vi "Control Panel Refresh.vi"(11 "Data In":string[][](array[string]) caption="所有行") -> (2 "Data":T1(array[cluster]), 3 "Array":cluster{string[][]}[](array[cluster]))   [LabVIEW 2020]
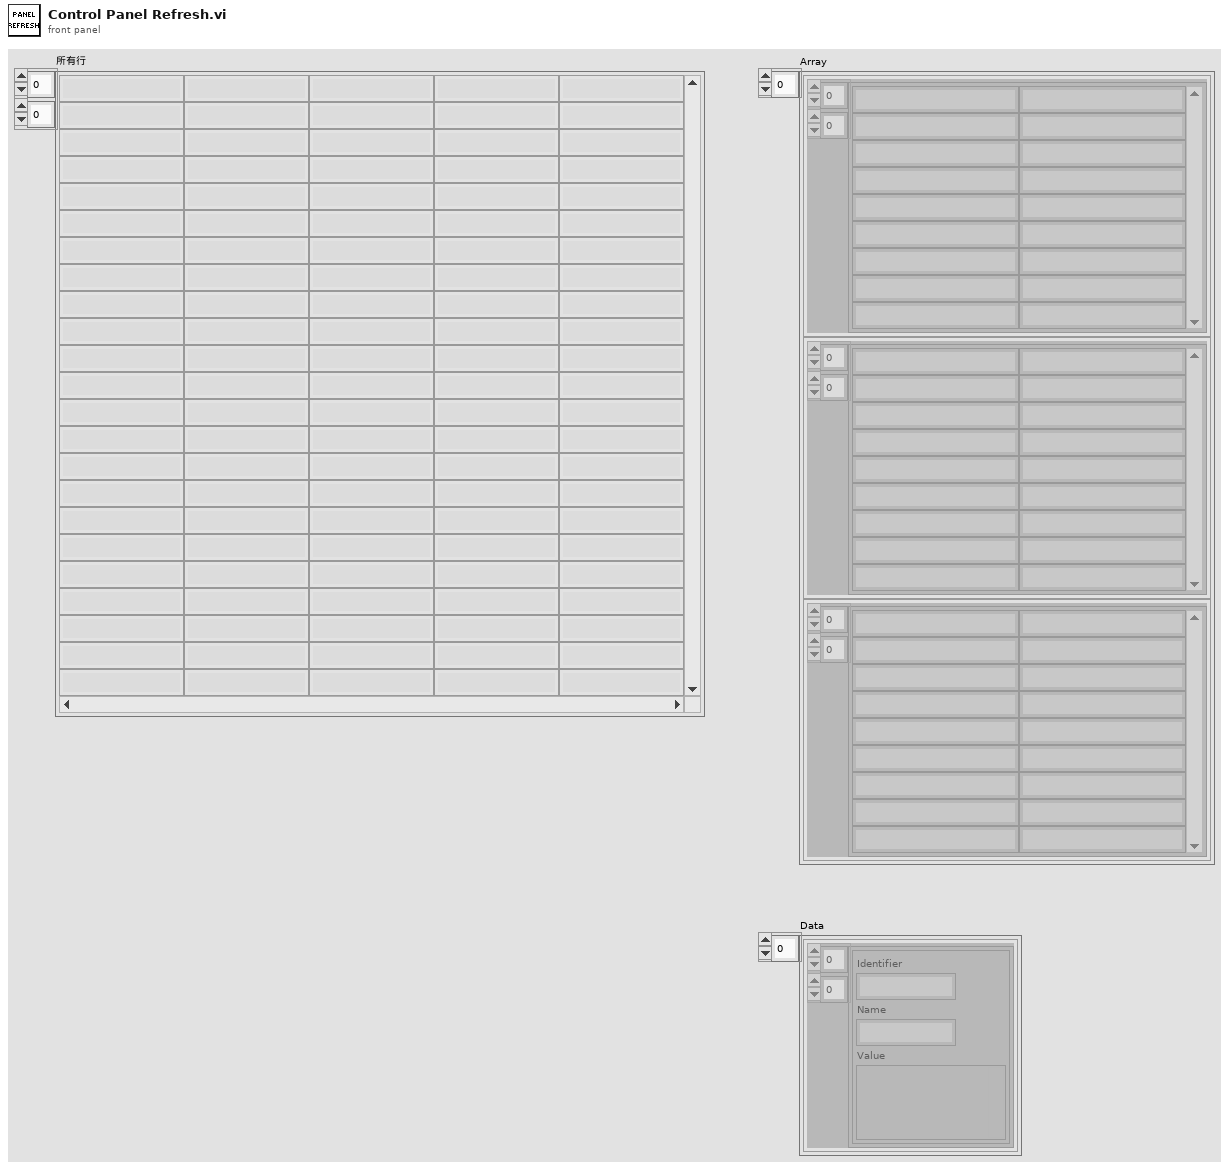
[diagram p1: front panel]
types:
  T1 = cluster{cluster{"Identifier":string, "Name":string, "Value":variant}[][]}[]
  T2 = map{string, map{string, cluster{"Module Name":string, "Name":string, "Index":string, "Identifier":string}}}
  T3 = map{string, cluster{"Module Name":string, "Name":string, "Index":string, "Identifier":string}}
  T4 = cluster{"Module Name":string, "Name":string, "Index":string, "Identifier":string}
  T5 = cluster{"Identifier":string, "Name":string, "Value":variant}
  T6 = cluster{"Identifier":string, "Name":string, "Value":variant}[]
  T7 = cluster{"Identifier":string, "Name":string, "Value":variant}[][]
  T8 = cluster{cluster{"Identifier":string, "Name":string, "Value":variant}[][]}
  T9 = typedef "LVRectTypeDef.ctl" = cluster{"Left":i16, "Top":i16, "Right":i16, "Bottom":i16}
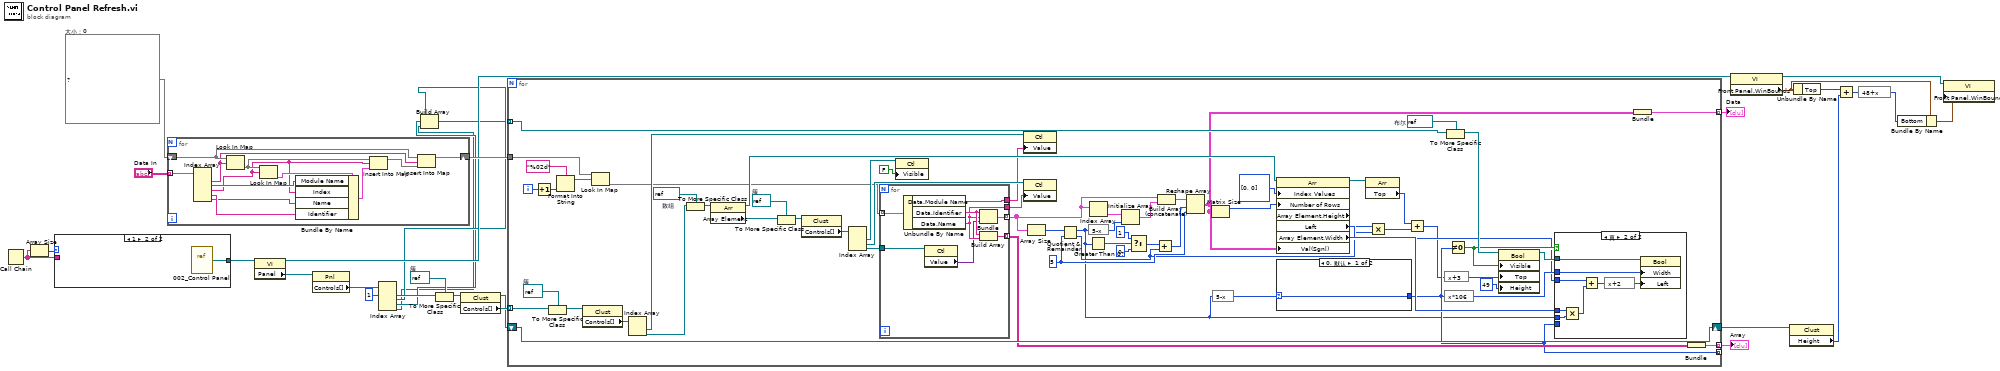
[diagram p0: block diagram]
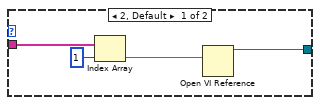
[diagram p4: hidden frame]
diagram:
  w19 = T2 {}  # 大小：0
  w24 = refnum<vi> refnum  # 簇
  n1 = Call Chain() -> (call chain=w28:string[])
  n2 = Array Size(array=w28) -> (size(s)=w29:i32)
  n3 = case shown="1" w29 {
    tunnel: w28 -> [w33 _]
    tunnel: [w30 w34] -> w27
    frame 2, Default {
      n4 = Index Array(array=w33, index=1 ("索引")) -> (element=w32:string)
      n5 = Open VI Reference(vi path=w32) -> (vi reference=w30:refnum<vi>)  [unwired: 5 in, 1 out]
    }
    frame 1 {
      n6 = vi-ref "002_Control Panel.vi"() -> (w34:refnum<vi>)
    }
  }
  n7 = for {
    tunnel: "Data In" -> [w44] mode=indexing
    shift-right: [w45] -> w18
    shift-left: w19 -> [w46]
    n8 = Index Array(array=w44) -> (element #1=w42:string, element #2=w38:string, element #3=w37:string, element #4=w36:string, element #5=w35:string)  [unwired: 5 in]
    n9 = Look In Map(map=w46, key=w42) -> (value=w41:T3)  [unwired: 1 in, 1 out]
    n10 = Look In Map(map=w41, key=w37) -> (value=w43:T4)  [unwired: 1 in, 1 out]
    n11 = Bundle By Name(cluster=w43, "Module Name"=w38, "Index"=w37, "Name"=w35, "Identifier"=w36) -> (w40:T4)
    n12 = Insert Into Map(map in=w41, key=w37, value=w40) -> (map out=w39:T3)  [unwired: 2 out]
    n13 = Insert Into Map(map in=w46, key=w42, value=w39) -> (map out=w45:T2)  [unwired: 2 out]
  }
  n14 = property class="VI"(reference=w27) -> (reference out=w17:refnum<vi>, "Panel"=w26:refnum<vi>)  [unwired: 1 in, 1 out]
  n15 = property class="Pnl"(reference=w26) -> ("Controls[]"=w25:refnum<vi>[])  [unwired: 1 in, 2 out]
  n16 = Index Array(array=w25, index #1=1 ("索引")) -> (element #1=w23:refnum<vi>, element #2=w5:refnum<vi>, element #3=w4:refnum<vi>, element #4=w3:refnum<vi>)  [unwired: 3 in]
  n17 = Build Array(w5, w4, w3) -> (w2:refnum<vi>[])
  n18 = To More Specific Class(target class=w24, reference=w23) -> (specific class reference=w22:refnum<vi>)  [unwired: 1 in, 1 out]
  n19 = property class="Clust"(reference=w22) -> (reference out=w10:refnum<vi>, "Controls[]"=w21:refnum<vi>[])  [unwired: 1 in, 1 out]
  n20 = for {
    tunnel: w21 -> [w109] mode=indexing
    tunnel: w18 -> [w54]
    shift-right: [w82] -> w9
    shift-left: w10 -> [w82]
    tunnel: [w80] -> w7 mode=indexing
    tunnel: w2 -> [w79] mode=indexing
    tunnel: [w68] -> _ mode=indexing
    tunnel: [w48] -> w1 mode=indexing
    i -> [w52]
    w77 = refnum<vi> refnum  # 布尔
    w88 = 5 ("y")
    w101 = refnum<vi> refnum  # 簇
    w104 = refnum<vi> refnum  # 数组
    w108 = refnum<vi> refnum  # 簇
    n21 = Increment(x=w52) -> (x+1=w51:i32)
    n22 = To More Specific Class(target class=w108, reference=w109) -> (specific class reference=w107:refnum<vi>)  [unwired: 1 in, 1 out]
    n23 = Format Into String(format string="%02d" ("格式字符串"), w51) -> (resulting string=w50:string)  [unwired: 2 in, 1 out]
    n24 = property class="Clust"(reference=w107) -> ("Controls[]"=w106:refnum<vi>[])  [unwired: 1 in, 2 out]
    n25 = Look In Map(map=w54, key=w50) -> (value=w49:T3)  [unwired: 1 in, 1 out]
    n26 = Index Array(array=w106) -> (element #1=w85:refnum<vi>, element #2=w103:refnum<vi>)  [unwired: 2 in]
    n27 = To More Specific Class(target class=w104, reference=w103) -> (specific class reference=w105:refnum<vi>)  [unwired: 1 in, 1 out]
    n28 = property class="Arr"(reference=w105) -> (reference out=w93:refnum<vi>, "Array Element"=w100:refnum<vi>)  [unwired: 1 in, 1 out]
    n29 = To More Specific Class(target class=w101, reference=w100) -> (specific class reference=w102:refnum<vi>)  [unwired: 1 in, 1 out]
    n30 = property class="Clust"(reference=w102) -> ("Controls[]"=w99:refnum<vi>[])  [unwired: 1 in, 2 out]
    n31 = Index Array(array=w99) -> (element #1=w98:refnum<vi>, element #2=w96:refnum<vi>, element #3=w95:refnum<vi>)  [unwired: 3 in]
    n32 = for {
      tunnel: w95 -> [w126]
      tunnel: [w121] -> w94
      tunnel: w49 -> [w125] mode=indexing
      tunnel: [w124] -> w58 mode=indexing
      tunnel: [w123] -> w84
      tunnel: [w120] -> w81 mode=indexing
      n33 = Unbundle By Name(w125) -> ("Data.Module Name"=w123:string, "Data.Identifier"=w122:string, "Data.Name"=w121:string)
      n34 = property class="Ctl"(reference=w126) -> ("Value"=w119:variant)  [unwired: 1 in, 2 out]
      n35 = Bundle("Identifier"=w122, "Name"=w121, "Value"=w119) -> (w124:T5)  [unwired: 1 in]
      n36 = Build Array(w122, w121) -> (w120:string[])
    }
    n37 = property class="Ctl"(reference=w98, "Visible"=FALSE ("可见")) -> ()  [unwired: 1 in, 2 out]
    n38 = property class="Ctl"(reference=w85, "Value"=w84) -> ()  [unwired: 1 in, 2 out]
    n39 = property class="Ctl"(reference=w96, "Value"=w94) -> ()  [unwired: 1 in, 2 out]
    n40 = Array Size(array=w58) -> (size(s)=w70:i32)
    n41 = Quotient & Remainder(x=w70, y=w88) -> (x-y*floor(x/y)=w61:i32, floor(x/y)=w66:i32)
    n42 = expression code="5-x"(w61) -> (w71:i32)
    n43 = Index Array(array=w58) -> (element=w87:T5)  [unwired: 1 in]
    n44 = Greater Than 0?(x=w61) -> (x > 0?=w90:bool)
    n45 = Initialize Array(w87, w71) -> (w57:T6)
    n46 = Select(t=1, s=w90, f=0) -> (s? t:f=w89:i32)
    n47 = Add(x=w89, y=w66) -> (x+y=w86:i32)
    n48 = Build Array (concatenate)(w58, w57) -> (w56:T6)
    n49 = Reshape Array(w56, w86, w88) -> (w47:T7)
    n50 = Matrix Size(0:w47) -> (1:w83:i32)  [unwired: 1 out]
    n51 = expression code="5-x"(w61) -> (w69:i32)
    n52 = property class="Arr"(reference=w93, "Index Values"=u32[] [0, 0] ("索引值"), "Number of Rows"=w83, "Val(Sgnl)"=w47) -> (reference out=w60:refnum<vi>, "Array Element.Height"=w65:u32, "Left"=w72:i32, "Array Element.Width"=w73:u32)  [unwired: 1 in, 1 out]
    n53 = case shown="0, 默认" w69 {
      selector: w69 -> [w110 _]
      tunnel: [w110 _] -> w68
      frame 0, Default {
      }
      frame 5.. {
      }
    }
    n54 = property class="Arr"(reference=w60) -> ("Top"=w59:i32)  [unwired: 1 in, 2 out]
    n55 = Multiply(x=w65, y=w66) -> (x*y=w64:u32)
    n56 = Add(x=w59, y=w64) -> (x+y=w63:u32)
    n57 = expression code="x*106"(w68) -> (w75:i32)
    n58 = expression code="x+3"(w63) -> (w62:u32)
    n59 = To More Specific Class(target class=w77, reference=w79) -> (specific class reference=w78:refnum<vi>)  [unwired: 1 in, 1 out]
    n60 = Not Equal To 0?(x=w68) -> (x != 0?=w74:bool)
    n61 = property class="Bool"(reference=w78, "Visible"=w74, "Top"=w62, "Height"=u32 49 ("按钮大小:高度")) -> (reference out=w76:refnum<vi>)  [unwired: 1 in, 1 out]
    n62 = case shown="真" w74 {
      tunnel: w76 -> [_ w118]
      tunnel: w75 -> [_ w117]
      tunnel: w68 -> [_ _]
      tunnel: w73 -> [_ w116]
      tunnel: w72 -> [_ w115]
      tunnel: w61 -> [_ w111]
      frame False {
      }
      frame True {
        n63 = Multiply(x=w116, y=w111) -> (x*y=w113:u32)
        n64 = Add(x=w115, y=w113) -> (x+y=w114:u32)
        n65 = expression code="x+2"(w114) -> (w112:u32)
        n66 = property class="Bool"(reference=w118, "Width"=w117, "Left"=w112) -> ()  [unwired: 1 in, 2 out]
      }
    }
    n67 = Bundle(w47) -> (w48:T8)  [unwired: 1 in]
    n68 = Bundle(w81) -> (w80:cluster{string[][]})  [unwired: 1 in]
  }
  "Array" <- w7
  "Data" <- w1
  n69 = property class="VI"(reference=w17) -> (reference out=w15:refnum<vi>, "Front Panel.WinBounds"=w14:T9)  [unwired: 1 in, 1 out]
  n70 = property class="Clust"(reference=w9) -> ("Height"=w13:u32)  [unwired: 1 in, 2 out]
  n71 = Unbundle By Name(w14) -> ("Top"=w12:i16)
  n72 = Add(x=w12, y=w13) -> (x+y=w11:u32)
  n73 = expression code="48+x"(w11) -> (w8:u32)
  n74 = Bundle By Name(cluster=w14, "Bottom"=w8) -> (w16:T9)
  n75 = property class="VI"(reference=w15, "Front Panel.WinBounds"=w16) -> ()  [unwired: 1 in, 2 out]
